vi "sir_v6.vi"() -> ()   [LabVIEW 2009]
panel:
  out "Restul sirului incepand cu sirul cautat":string="Inginerie Electrica"
  in  "Sirul 2":string="Inginerie "
  out "Pozitia de incepiut a sirului cautat":dbl=11.0
  in  "stop":bool
  out "Sirul din fata":string="Catedra de "
  in  "Sirul 1":string="Catedra de Inginerie Electrica"
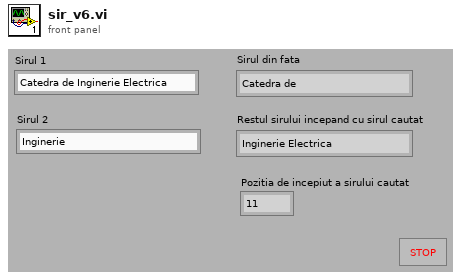
[diagram p1: front panel]
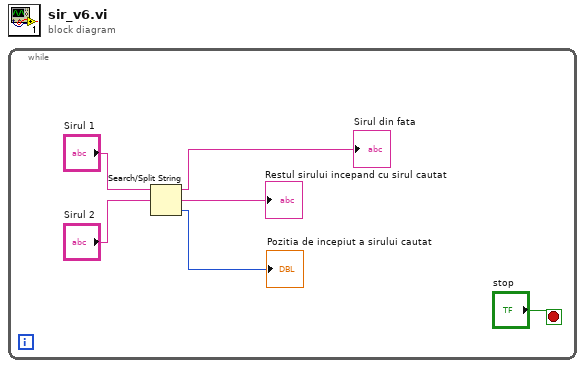
[diagram p0: block diagram]
diagram:
  n1 = while {
    stop <- "stop" stop-if-true
    n2 = Search/Split String(string="Sirul 1", search string/char (-)="Sirul 2") -> (substring before match=→"Sirul din fata":string, match + rest of string=→"Restul sirului incepand cu sirul cautat":string, offset of match=→"Pozitia de incepiut a sirului cautat":i32)  [unwired: 1 in]
  }
